vi "Overview Get Overview Limit.vi"(8 "error in":errorcluster, 11 "XYGraphOverview in":refnum<class "XYGraphOverview.lvclass">) -> (0 "error out":errorcluster, 2 "Limit":cluster{"Lower Limit":dbl, "Upper Limit":dbl}, 3 "XYGraphOverview out":refnum<class "XYGraphOverview.lvclass">)   [LabVIEW 2020, in "XYGraphOverview.lvlib" / "XYGraphOverview.lvclass"]
uses:
  XYGraphOverview.lvclass
  XYGraphOverview.lvclass/XYGraphOverview.ctl
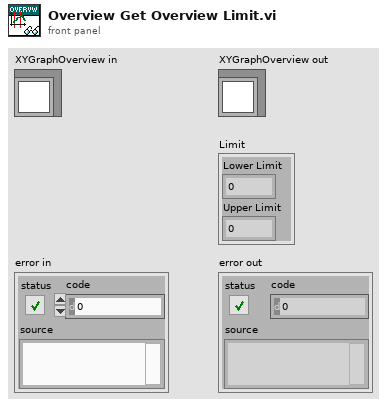
[diagram p1: front panel]
types:
  T1 = cluster{"Cursor.Cursor X":dbl, "Cursor.Cursor X":dbl}
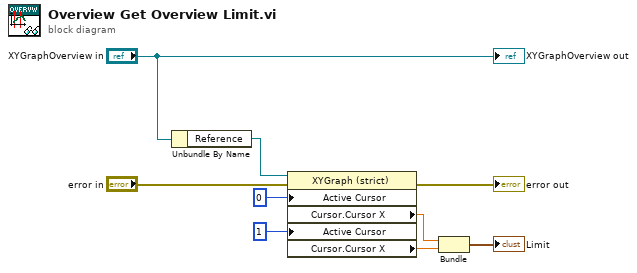
[diagram p0: block diagram]
diagram:
  n1 = Unbundle By Name("XYGraphOverview in") -> ("Reference"=w1:refnum<vi>)
  n2 = property on="Property Node" class="XYGraph (strict)"(reference=w1, error in="error in", "Active Cursor"=u32 0, "Active Cursor"=u32 1) -> (error out=→"error out":errorcluster, "Cursor.Cursor X"=w4:dbl, "Cursor.Cursor X"=w5:dbl)  [unwired: 1 out]
  n3 = Bundle("Cursor.Cursor X"=w4, "Cursor.Cursor X"=w5) -> (→"Limit":T1)  [unwired: 1 in]
  "XYGraphOverview out" <- "XYGraphOverview in"
